vi "To String.vi"(8 "error in (no error)":errorcluster, 11 "Double Array in":refnum<class "Double Array.lvclass">) -> (0 "error out":errorcluster, 2 "String":string)   [LabVIEW 2020, in "Data.lvlib" / "Double Array.lvclass"]
doc: "Convert 'Generic Data in' to a string."
uses:
  Double Array.lvclass
  Double Array.lvclass/Double Array.ctl
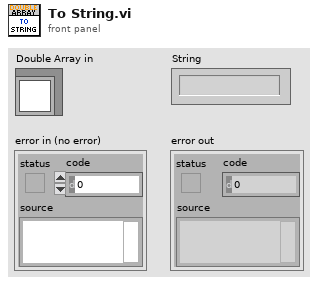
[diagram p1: front panel]
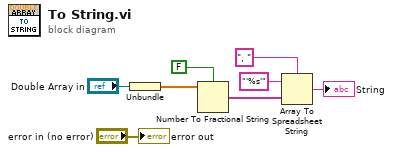
[diagram p0: block diagram]
diagram:
  n1 = Unbundle("Double Array in") -> (w3:dbl[])
  n2 = Number To Fractional String(use system decimal point (T)=FALSE, number=w3) -> (F-format string=w2:string[])  [unwired: 2 in]
  n3 = Array To Spreadsheet String(delimiter (Tab)=", ", array=w2, 3:"'%s'" ("format string")) -> (spreadsheet string=→"String":string)
  "error out" <- "error in (no error)"
